vi "Simple sin wave generator.vi"() -> ()   [LabVIEW 2023]
uses:
  <vilib>/measure/NI_MABase.lvlib
panel:
  out "I/P Frequency Value":dbl
  in  "Step Value":dbl=10.0
  out "Number of steps":dbl=nan
  in  "Starting frequency":dbl=1000.0
  in  "Ending frequency":dbl=2000.0
  in  "sampling info":cluster{"Fs":dbl, "#s":dbl}={"Fs"=1000.0, "#s"=1000.0} {"Fs" format="%.2p"}
  out "dt":dbl
  out "Samples":i32
  out "Waveform Graph":waveform(dbl)(graph)
  in  "phase":dbl(knob) scale=0.0..10.0
  in  "amplitude":dbl=1.0
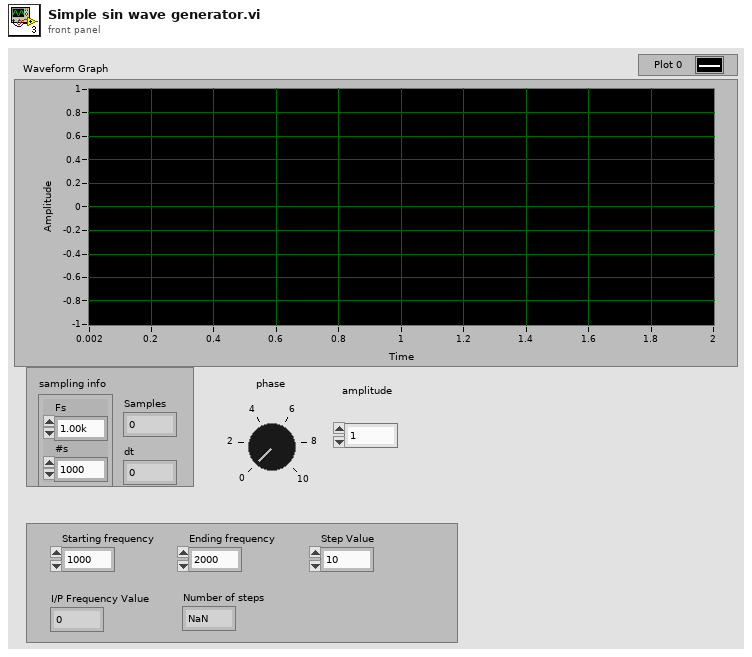
[diagram p1: front panel]
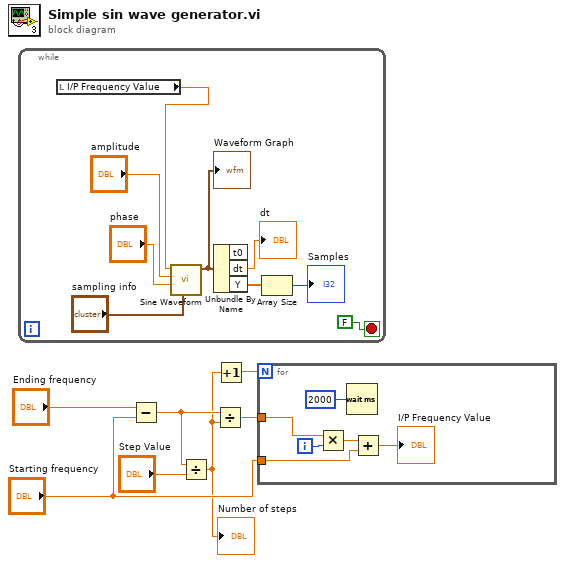
[diagram p0: block diagram]
diagram:
  n1 = while {
    stop <- FALSE stop-if-true
    n2 = local read "I/P Frequency Value"() -> (w8:dbl)
    n3 = call <vilib>:"Sine Waveform.vi"("sampling info"="sampling info", "phase"="phase", "amplitude"="amplitude", "frequency"=w8) -> ("signal out"=w14:waveform(dbl))  [unwired: 6 in, 1 out]
    "Waveform Graph" <- w14
    n4 = Unbundle By Name(w14) -> ("dt"=→"dt":dbl, "Y"=w13:dbl[])  [unwired: 1 out]
    n5 = Array Size(array=w13) -> (size(s)=→"Samples":i32)
  }
  n6 = Subtract(x="Ending frequency", y="Starting frequency") -> (x-y=w3:dbl)
  n7 = Divide(x=w3, y="Step Value") -> (x/y=w1:dbl)
  "Number of steps" <- w1
  n8 = Divide(x=w3, y=w1) -> (x/y=w6:dbl)
  n9 = Increment(x=w1) -> (x+1=w4:dbl)
  n10 = for {
    N: w4 -> [_]
    tunnel: w6 -> [w22]
    tunnel: "Starting frequency" -> [w19]
    i -> [w21]
    n11 = Multiply(x=w22, y=w21) -> (x*y=w20:dbl)
    n12 = Wait (ms)(milliseconds to wait=u32 2000) -> ()  [unwired: 1 out]
    n13 = Add(x=w20, y=w19) -> (x+y=→"I/P Frequency Value":dbl)
  }
